vi "Get Size.vi"(8 "error in (no error)":errorcluster, 11 "Transfer Runtime in":refnum<class "Runtime.Transfer.lvclass">) -> (0 "error out":errorcluster, 2 "size in bytes":u64, 3 "Transfer Runtime out":refnum<class "Runtime.Transfer.lvclass">)   [LabVIEW 2016, in "Data Sharing Framework.Runtime.lvlib" / "Runtime.Transfer.lvclass"]
uses:
  Runtime.Transfer.lvclass
  Runtime.Transfer.lvclass/Runtime.Transfer.ctl
  Channel/Runtime.Channel.lvclass
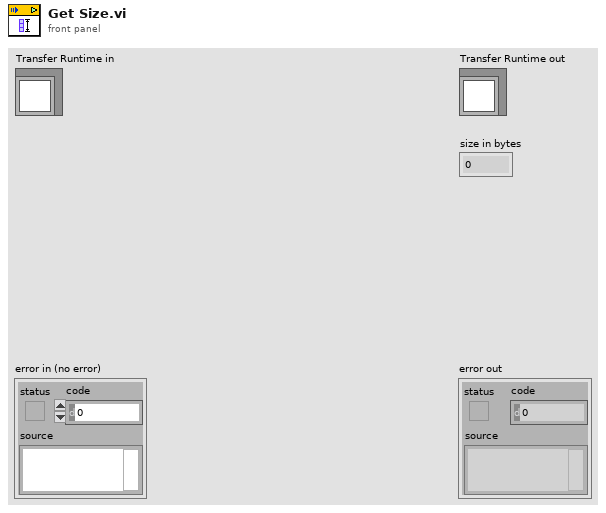
[diagram p1: front panel]
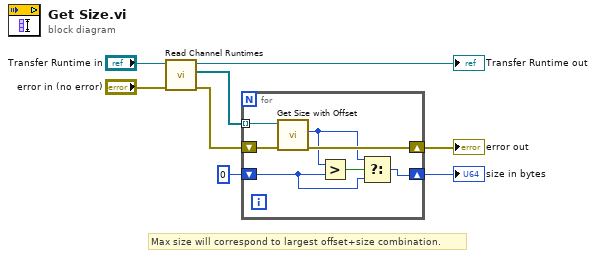
[diagram p0: block diagram]
diagram:
  # "Max size will correspond to largest offset+size combination."
  n1 = call "Read Channel Runtimes.vi"("error in (no error)"="error in (no error)", "Runtime.Transfer in"="Transfer Runtime in") -> ("error out"=w4:errorcluster, "Channel Runtimes"=w5:refnum<class "Runtime.Channel.lvclass">[], "Runtime.Transfer out"=→"Transfer Runtime out":refnum<class "Runtime.Transfer.lvclass">)  [unwired: 7 in]
  n2 = for {
    tunnel: w5 -> [w9] mode=indexing
    shift-right: [w11] -> w2
    shift-left: w4 -> [w12]
    shift-right: [w13] -> w1
    shift-left: u64 0 -> [w14]
    n3 = call "Get Size with Offset.vi"("error in (no error)"=w12, "Channel Runtime in"=w9) -> ("error out"=w11:errorcluster, "size+offset in bytes"=w10:u64)  [unwired: 7 in, 1 out]
    n4 = Greater?(x=w10, y=w14) -> (0:w15:bool)
    n5 = Select(t=w10, s=w15, f=w14) -> (s? t:f=w13:u64)
  }
  "error out" <- w2
  "size in bytes" <- w1
